vi "ModFileName.vi"() -> ()   [LabVIEW 2022 SP3]
panel:
  in  "Choose Write Directory":path
  in  "file ext":string="*.eye"
  in  "Use Selected Files":bool
  in  "Listbox":i32[](listbox)
  in  "Choose Read Directory":path
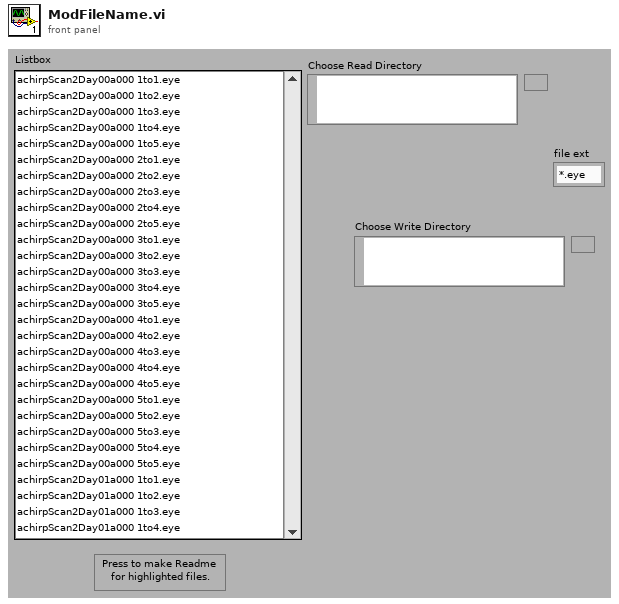
[diagram p1: front panel]
types:
  T1 = cluster{"organ":i16, "disease type":i16, "disease location":i16}
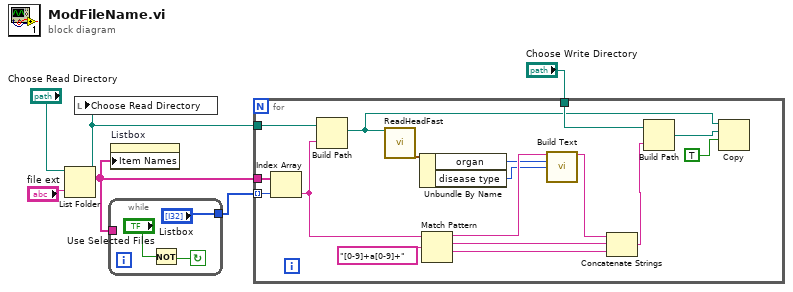
[diagram p0: block diagram]
diagram:
  n1 = List Folder(path="Choose Read Directory", pattern="file ext") -> (path out=w3:path, filenames=w6:string[])  [unwired: 1 in, 3 out]
  n2 = local write "Choose Read Directory"(w3) -> ()
  n3 = while {
    tunnel: ["Listbox"] -> w5
    tunnel: w6 -> [_]
    stop <- w9 continue-if-true
    n4 = Not(x="Use Selected Files") -> (.not. x?=w9:bool)
  }
  n5 = property on="Listbox" class="LstBox (strict)"("Item Names"=w6) -> ()  [unwired: 2 in, 2 out]
  n6 = for {
    tunnel: w6 -> [w26]
    tunnel: w5 -> [w25] mode=indexing
    tunnel: w3 -> [w18]
    tunnel: "Choose Write Directory" -> [w17]
    n7 = Index Array(array=w26, index=w25) -> (element=w22:string)
    n8 = Build Path(base path=w18, name or relative path=w22) -> (appended path=w16:path)
    n9 = call "ReadHeadFast.vi"("new file path"=w16) -> ("Tissue Type"=w24:T1)  [unwired: 2 in, 16 out]
    n10 = Unbundle By Name(w24) -> ("organ"=w20:i16, "disease type"=w19:i16)
    n11 = Match Pattern(string=w22, regular expression="[0-9]+a[0-9]+") -> (before substring=w21:string, match substring=w11:string, after substring=w10:string)  [unwired: 1 in, 1 out]
    n12 = call "Build Text"("Beginning Text"=w21, "p"=w20, "rf"=w19) -> ("Result"=w13:string)  [unwired: 11 in, 1 out]
    n13 = Concatenate Strings(w13, w11, w10) -> (w12:string)
    n14 = Build Path(base path=w17, name or relative path=w12) -> (appended path=w15:path)
    n15 = Copy(9:TRUE ("overwrite (F)"), 10:w15, 11:w16) -> ()  [unwired: 2 in, 3 out]
  }
